vi "setStage.vi"(8 "error in (no error)":errorcluster, 11 "ActionEditor in":refnum<class "ActionEditor.lvclass">) -> (0 "error out":errorcluster, 3 "ActionEditor out":refnum<class "ActionEditor.lvclass">)   [LabVIEW 2009, in "Views.lvlib" / "ScriptEditor.lvlib" / "ActionEditor.lvclass"]
uses:
  ActionEditor.lvclass
  ActionEditor.lvclass/ActionEditor.ctl
  Tools/Scripting/ScriptingEvent/ScriptEvent.lvclass
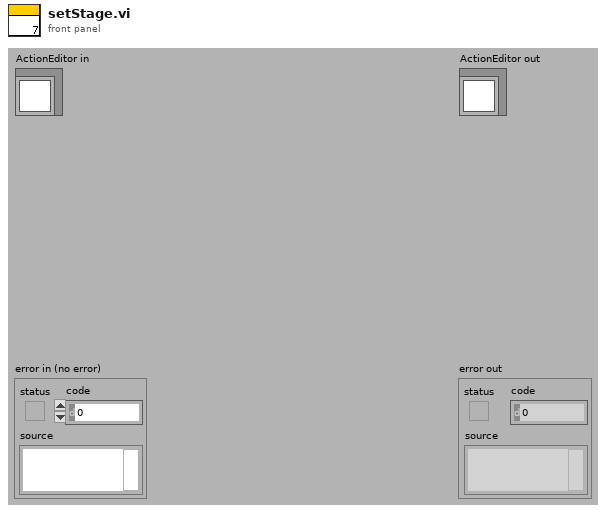
[diagram p1: front panel]
types:
  T1 = enum16{"Initialise", "MOT", "Molasses", "Optical Pumping", "Magnetic Trap", "RF Cooling", "Manipulation", "Switch Off", "Absorption Imaging", "Fluorscence Imaging", "Shut Down"}
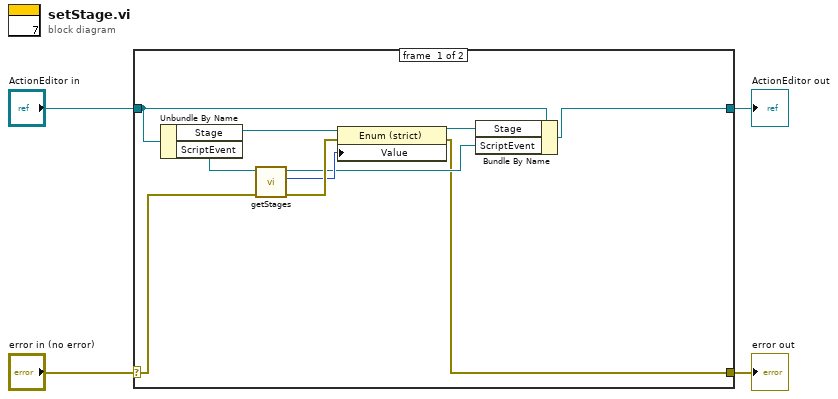
[diagram p0: block diagram]
diagram:
  n1 = case shown="No Error" "error in (no error)" {
    selector: "error in (no error)" -> [w13 w16]
    tunnel: [w5 w16] -> w3
    tunnel: [w7 w15] -> w1
    tunnel: "ActionEditor in" -> [w8 w15]
    frame #0 {
      n2 = Unbundle By Name(w8) -> ("Stage"=w12:refnum<vi>, "ScriptEvent"=w14:refnum<class "ScriptEvent.lvclass">)
      n3 = call "getStages.vi"("error in (no error)"=w13, "ScriptEvent.lvclass in"=w14) -> ("error out"=w11:errorcluster, "Stage"=w10:T1, "ScriptEvent.lvclass out"=w6:refnum<class "ScriptEvent.lvclass">)  [unwired: 7 in]
      n4 = property class="Enum (strict)"(reference=w12, error in=w11, "Value"=w10) -> (reference out=w9:refnum<vi>, error out=w5:errorcluster)
      n5 = Bundle By Name(cluster=w8, "Stage"=w9, "ScriptEvent"=w6) -> (w7:refnum<class "ActionEditor.lvclass">)
    }
    frame #1 {
    }
  }
  "error out" <- w3
  "ActionEditor out" <- w1
